vi "Create SSL Client Socket New.vi"() -> ()   [LabVIEW 2013, in "OpenSSL Socket.lvlib" / "SSL Client Context.lvclass"]
uses:
  SSL Client Context.lvclass
  SSL Client Socket/SSL Client Socket.lvclass
panel:
  out "error out":errorcluster
  in  "error in (no error)":errorcluster
  out "OpenSSL Socket.lvlib:SSL Client Skt":refnum<class "SSL Client Socket.lvclass">
  in  "OpenSSL Socket.lvlib:SSL Client Ctx":refnum<class "SSL Client Context.lvclass">
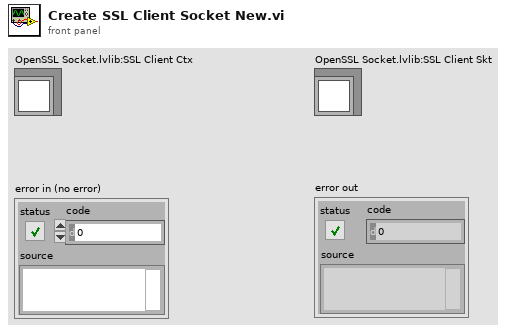
[diagram p1: front panel]
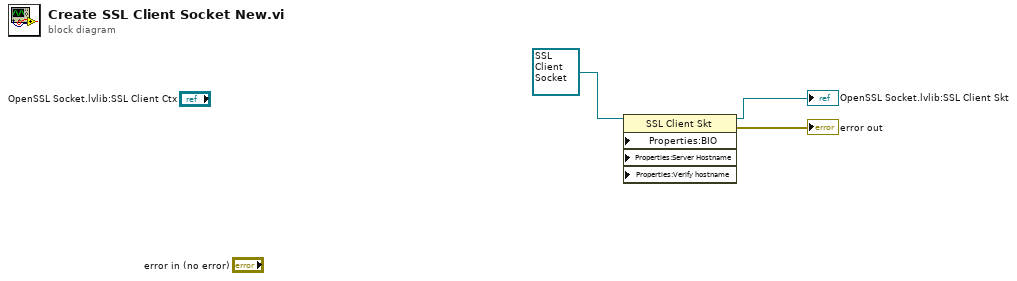
[diagram p0: block diagram]
diagram:
  n1 = property class="SSL Client Skt" props=["Properties:BIO", "Properties:Server Hostname", "Properties:Verify hostname"](reference=refnum<class "SSL Client Socket.lvclass"> refnum ("OpenSSL Socket.lvlib:SSL Client Skt")) -> (reference out=→"OpenSSL Socket.lvlib:SSL Client Skt":refnum<class "SSL Client Socket.lvclass">, error out=→"error out":errorcluster)  [unwired: 4 in]
